vi "Read Device Data.vi"(8 "error in (no error)":errorcluster, 11 "SLL in":refnum<class "SLL.lvclass">) -> (0 "error out":errorcluster, 2 "Device Data":string[][](array[string]), 3 "SLL out":refnum<class "SLL.lvclass">)   [LabVIEW 2023, in "SLL.lvlib" / "SLL.lvclass"]
uses:
  SLL.lvclass
  SLL.lvclass/SLL.ctl
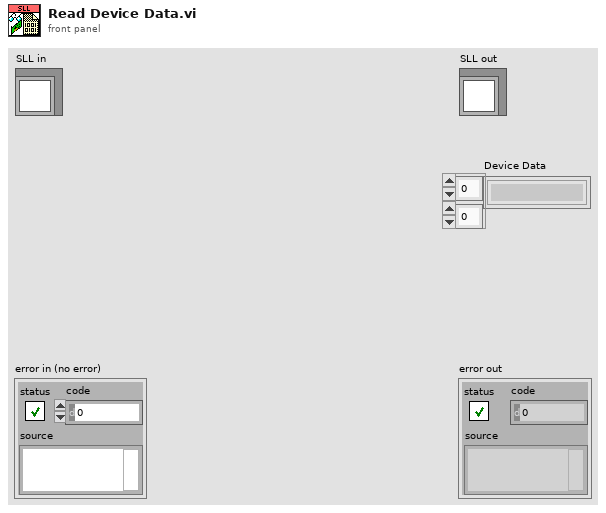
[diagram p1: front panel]
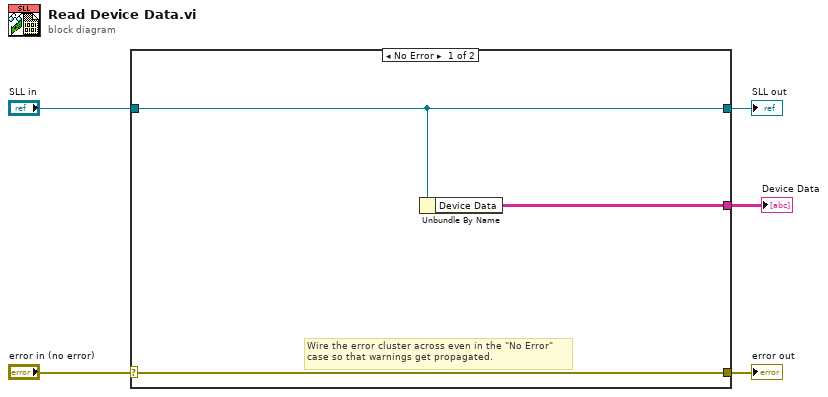
[diagram p0: block diagram]
diagram:
  n1 = case shown="No Error" "error in (no error)" {
    selector: "error in (no error)" -> [w8 w10]
    tunnel: [w8 w10] -> w4
    tunnel: [w7 w9] -> w2
    tunnel: "SLL in" -> [w7 w9]
    tunnel: [w6 _] -> w1
    frame No Error {
      # "Wire the error cluster across even in the \"No Error\"\ncase so that warnings get propagated."
      n2 = Unbundle By Name(w7) -> ("Device Data"=w6:string[][])
    }
    frame Error {
    }
  }
  "error out" <- w4
  "SLL out" <- w2
  "Device Data" <- w1
